vi "PicoScope6000aGetRapidBlockBulk.vi"(0 "handle in":i16, 1 "Acquisition Settings":T3 {"postTriggerSamples" format="%_6p"; "preTriggerSamples" format="%_6p"}, 2 "Buffer and Transfer Settings":T2 {"Down-Sample Mode" items=["None", "Aggregate", "Decimate", "Average"]; "Down Sample Ratio" step=1; "noOfSamples" format="%_6p"}, 3 "enabled array":i16[](array[numeric]), 7 "stop IsReady":bool, 11 "error in (no error)":errorcluster) -> (4 "handle out":i16, 6 "Buffers (Max or non-aggregated)":T1, 10 "Min Buffers":T1, 12 "noOfSamples":u64, 13 "nMaxSamples":u64, 14 "overflow":i16[](array[numeric]) format="%08b", 15 "error out":errorcluster)   [LabVIEW 2009]
doc: "This VI gets a set of blocks captured using rapid block mode. It outputs two-dimensional arrays for each channel that contain data from all the requested captures."
uses:
  ps6000a.dll
panel:
  in  "PicoAction 2":u32(ring) items=["NONE", "CLEAR_ALL", "ADD", "CLEAR_THIS_DATA_BUFFER", "CLEAR_WAVEFORM_DATA_BUFFERS", "CLEAR_WAVEFORM_READ_DATA_BUFFERS"]
  in  "PicoAction 1":u32(ring) items=["NONE", "CLEAR_ALL", "ADD", "CLEAR_THIS_DATA_BUFFER", "CLEAR_WAVEFORM_DATA_BUFFERS", "CLEAR_WAVEFORM_READ_DATA_BUFFERS"]
  # "Pico Buffer Actions"
  # "Samples can be equal to or less\nTotal Pre and Post Trigger Samples"
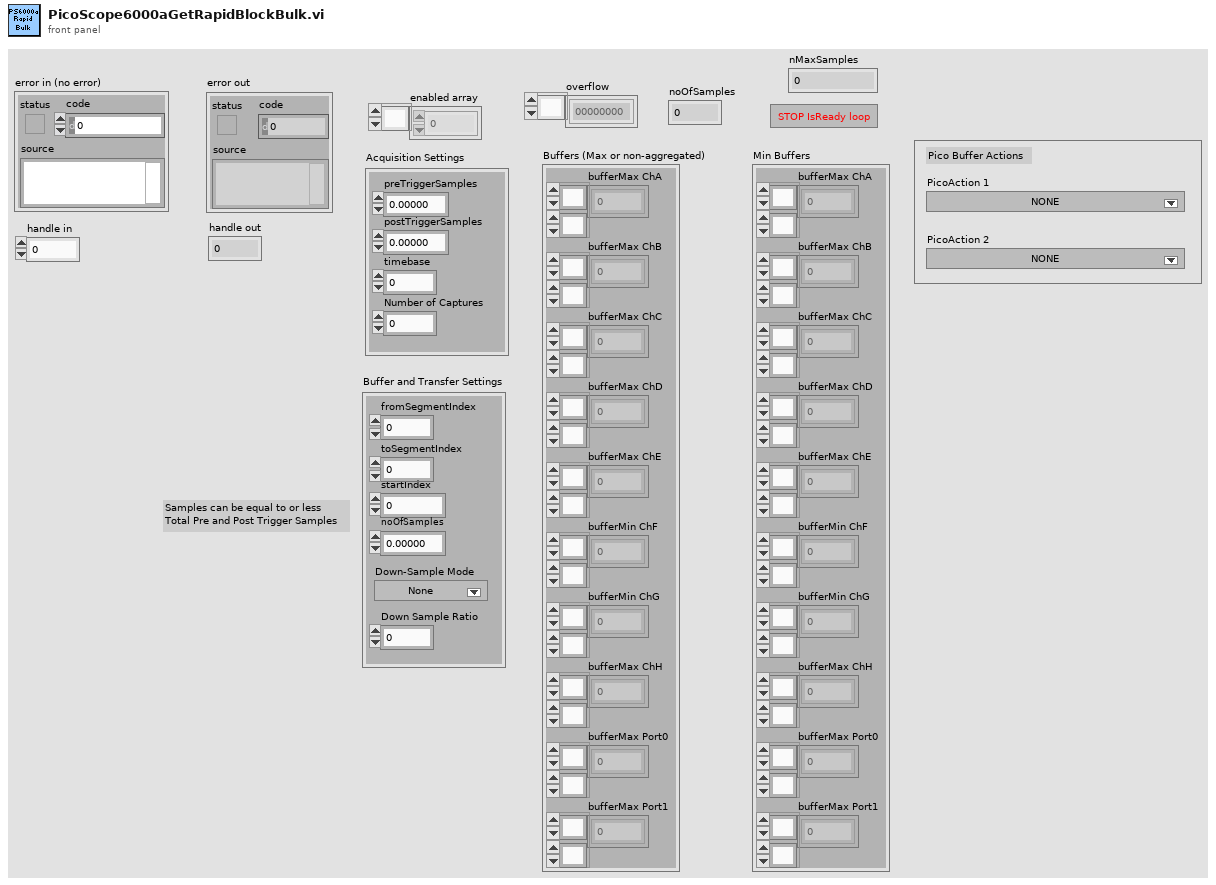
[diagram p1: front panel]
types:
  T1 = cluster{"bufferMax ChA":i16[][], "bufferMax ChB":i16[][], "bufferMax ChC":i16[][], "bufferMax ChD":i16[][], "bufferMax ChE":i16[][], "bufferMin ChF":i16[][], "bufferMin ChG":i16[][], "bufferMax ChH":i16[][], "bufferMax Port0":i16[][], "bufferMax Port1":i16[][]}
  T2 = cluster{"fromSegmentIndex":u64, "toSegmentIndex":u64, "startIndex":u64, "noOfSamples":u64, "Down-Sample Mode":u32, "Down Sample Ratio":u64}
  T3 = cluster{"preTriggerSamples":u64, "postTriggerSamples":u64, "timebase":u32, "Number of Captures":u64}
  T4 = enum32{"PICO_INT8_T", "PICO_INT16_T", "PICO_INT32_T", "PICO_UINT32_T", "PICO_INT64_T", ""}
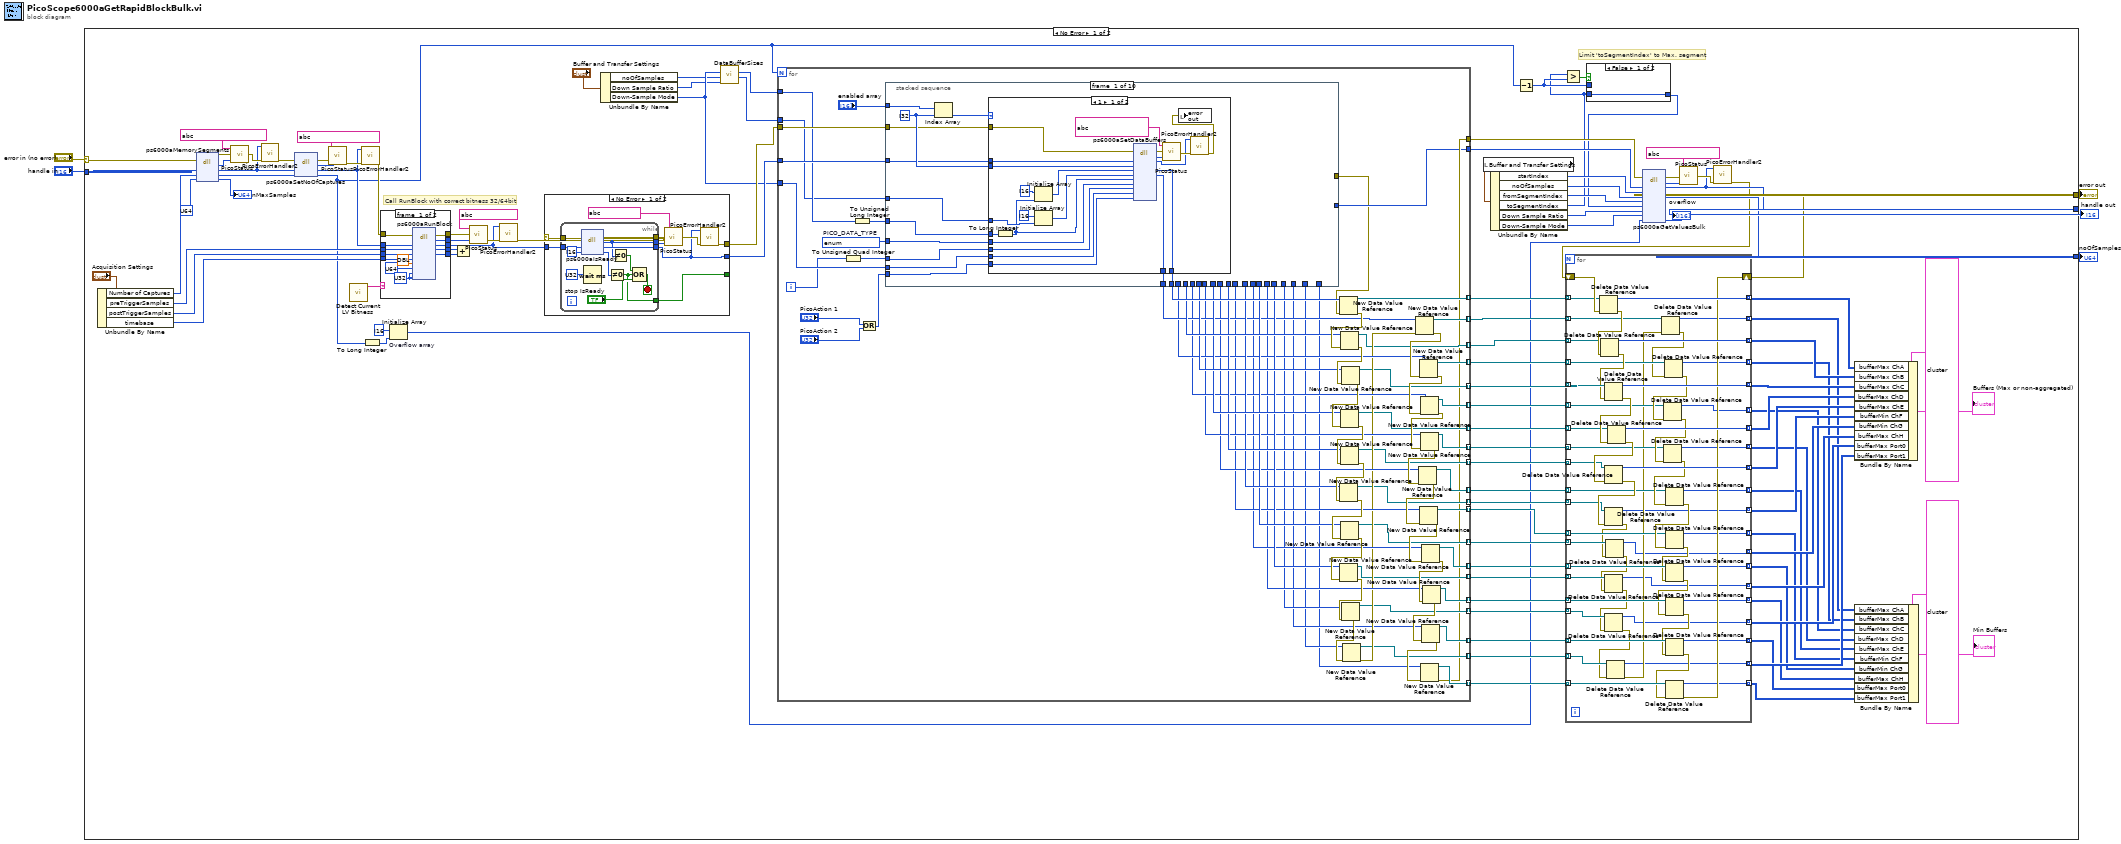
[diagram p0: block diagram]
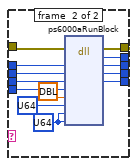
[diagram p2: hidden frame]
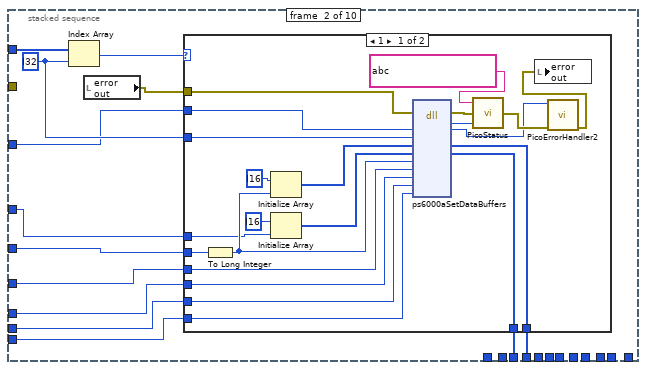
[diagram p5: hidden frame]
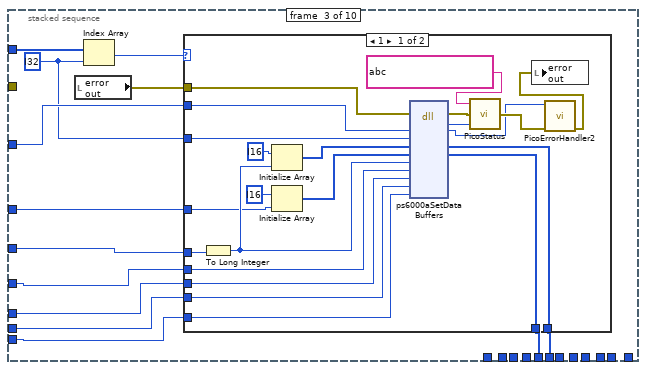
[diagram p7: hidden frame]
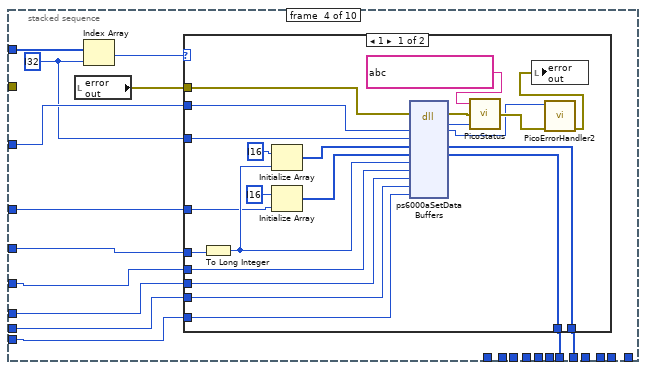
[diagram p9: hidden frame]
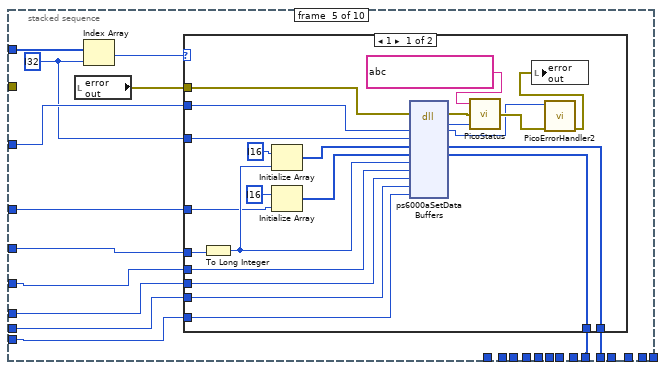
[diagram p11: hidden frame]
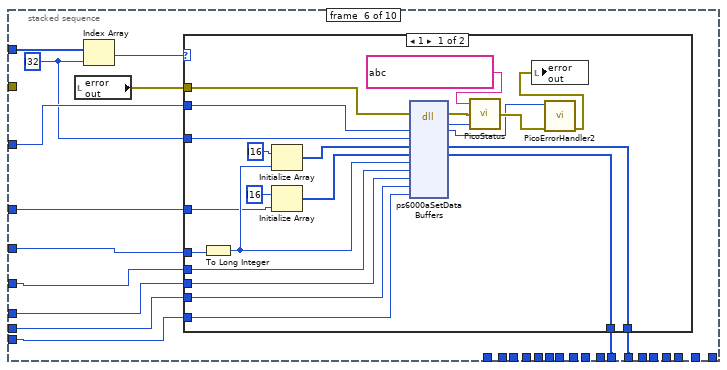
[diagram p13: hidden frame]
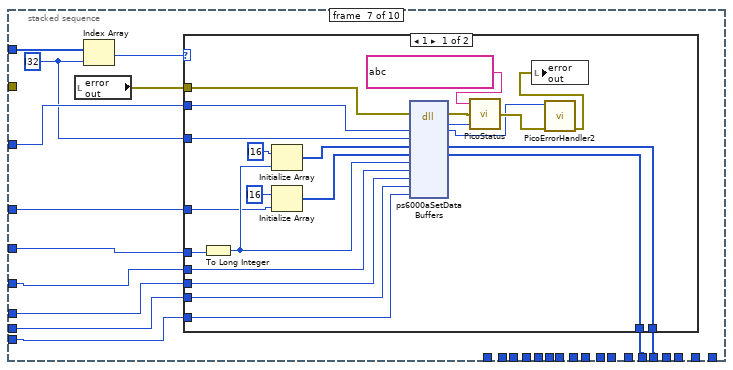
[diagram p15: hidden frame]
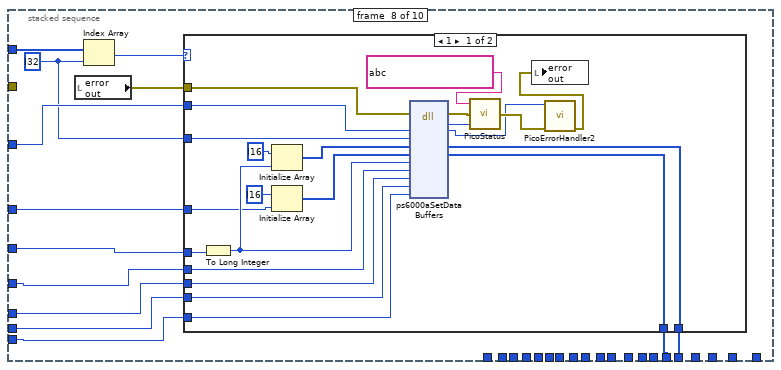
[diagram p17: hidden frame]
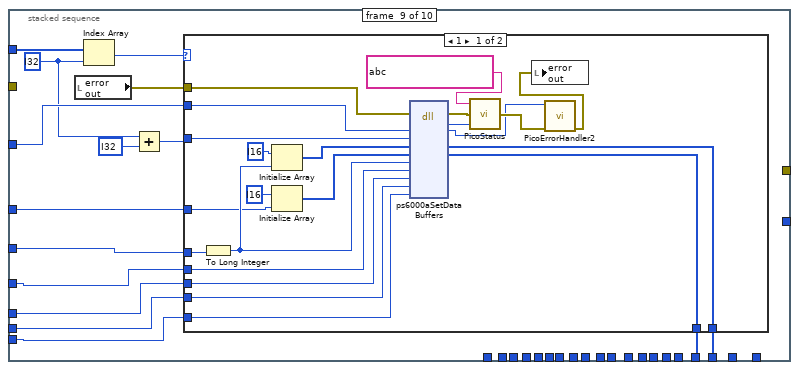
[diagram p19: hidden frame]
diagram:
  n1 = case shown="No Error" "error in (no error)" {
    selector: "error in (no error)" -> [w79 w662]
    tunnel: [w53 w662] -> w5
    tunnel: "handle in" -> [w78 w661]
    tunnel: [w75 w661] -> w4
    tunnel: [w103 u32 ? ("noOfSamples")] -> w1
    frame #0 {
      # "Call RunBlock with correct bitness 32/64bit"
      # "Limit 'toSegmentIndex' to Max. segment"
      n2 = Unbundle By Name("Acquisition Settings") -> ("Number of Captures"=w80:u64, "preTriggerSamples"=w107:u64, "postTriggerSamples"=w106:u64, "timebase"=w105:u32)
      n3 = dll-call lib="ps6000a.dll" fn="ps6000aMemorySegments" ("ps3000.dll:_ps3000_open_unit@0")(error in=w79, "handle"=w78, "nSegments"=w80, "nMaxSamples"=u64 ?) -> (error out=w91:errorcluster, "PICO_STATUS"=w92:u32, "handle"=w84:i16, "nSegments"=w88:u64, "nMaxSamples"=→"nMaxSamples":u64)  [unwired: 2 in, 1 out]
      n4 = call "PicoStatus.vi"("PICO STATUS"=w92, "error in"=w91, "source"=string ?) -> ("error out"=w85:errorcluster)
      n5 = call "PicoErrorHandler2.vi"("error in (no error)"=w85, "handle In"=w84) -> ("error out"=w11:errorcluster)  [unwired: 9 in]
      n6 = dll-call lib="ps6000a.dll" fn="ps6000aSetNoOfCaptures" ("ps3000.dll:_ps3000_open_unit@0")(error in=w11, "handle"=w84, "nCaptures"=w88) -> (error out=w87:errorcluster, "PICO_STATUS"=w82:u32, "handle"=w76:i16, "nCaptures"=w17:u64)  [unwired: 2 in, 1 out]
      n7 = call "PicoStatus.vi"("PICO STATUS"=w82, "error in"=w87, "source"=string ?) -> ("error out"=w83:errorcluster)
      n8 = call "Detect Current LV Bitness.vi"() -> ("bitness"=w12:string)  [unwired: 11 in]
      n9 = call "PicoErrorHandler2.vi"("error in (no error)"=w83, "handle In"=w76) -> ("error out"=w77:errorcluster)  [unwired: 9 in]
      n10 = To Long Integer(number=w17) -> (32bit integer=w25:i32)
      n11 = case shown="\"64\"" w12 {
        tunnel: [w126 w139] -> w113
        tunnel: [w125 w138] -> w112
        tunnel: [w124 w137] -> w110
        tunnel: [w123 w136] -> w109
        tunnel: w107 -> [w121 w134]
        tunnel: w106 -> [w120 w133]
        tunnel: w105 -> [w119 w132]
        tunnel: [w118 w131] -> w99
        tunnel: w77 -> [w116 w129]
        tunnel: w76 -> [w115 w128]
        frame #0 {
          w117 = u32 ? ("pParameter")
          n12 = dll-call lib="ps6000a.dll" fn="ps6000aRunBlock" ("ps3000.dll:_ps3000_open_unit@0")(error in=w116, "handle"=w115, "noOfPreTriggerSamples"=w121, "noOfPostTriggerSamples"=w120, "timebase"=w119, "timeIndisposedMs"=dbl ? ("pParameter"), "segmentIndex"=u64 ?, "lpReady"=w117, "pParameter"=w117) -> (error out=w123:errorcluster, "PICO_STATUS"=w124:u32, "handle"=w118:i16, "noOfPreTriggerSamples"=w126:u64, "noOfPostTriggerSamples"=w125:u64)  [unwired: 7 in, 1 out]
        }
        frame #1 {
          w130 = u64 ? ("pParameter")
          n13 = dll-call lib="ps6000a.dll" fn="ps6000aRunBlock" ("ps3000.dll:_ps3000_open_unit@0")(error in=w129, "handle"=w128, "noOfPreTriggerSamples"=w134, "noOfPostTriggerSamples"=w133, "timebase"=w132, "timeIndisposedMs"=dbl ? ("pParameter"), "segmentIndex"=u64 ?, "lpReady"=w130, "pParameter"=w130) -> (error out=w136:errorcluster, "PICO_STATUS"=w137:u32, "handle"=w131:i16, "noOfPreTriggerSamples"=w139:u64, "noOfPostTriggerSamples"=w138:u64)  [unwired: 7 in, 1 out]
        }
      }
      n14 = Initialize Array "Overflow array"(i16 ? ("element"), w25) -> (w24:i16[])
      n15 = Add(x=w113, y=w112) -> ()  [unwired: 1 out]
      n16 = call "PicoStatus.vi"("PICO STATUS"=w110, "error in"=w109, "source"=string ?) -> ("error out"=w104:errorcluster)
      n17 = call "PicoErrorHandler2.vi"("error in (no error)"=w104, "handle In"=w99) -> ("error out"=w102:errorcluster)  [unwired: 9 in]
      n18 = case shown="No Error" w102 {
        selector: w102 -> [w643 w658]
        tunnel: w99 -> [w644 w659]
        tunnel: [w637 w659] -> w100
        tunnel: [w638 w658] -> w101
        tunnel: [w636 bool ?] -> _
        frame #0 {
          n19 = while {
            tunnel: [w656] -> w637
            tunnel: w644 -> [w655]
            tunnel: [w652] -> w641
            tunnel: w643 -> [w651]
            tunnel: [w650] -> w642
            tunnel: [w645] -> w636
            stop <- w654 stop-if-true
            n20 = dll-call lib="ps6000a.dll" fn="ps6000aIsReady" ("ps3000.dll:_ps3000_open_unit@0")(error in=w651, "handle"=w655, "ready"=i16 ?) -> (error out=w650:errorcluster, "PICO_STATUS"=w652:u32, "handle"=w656:i16, "ready"=w646:i16)  [unwired: 2 in, 1 out]
            n21 = Wait (ms)(milliseconds to wait=u32 ?) -> ()  [unwired: 1 out]
            n22 = Not Equal To 0?(x=w646) -> (x != 0?=w645:bool)
            n23 = Not Equal To 0?(x=w652) -> (x != 0?=w653:bool)
            n24 = Compound Arithmetic op=OR(w653, w645, "stop IsReady") -> (w654:bool)
          }
          n25 = call "PicoStatus.vi"("PICO STATUS"=w641, "error in"=w642, "source"=string ?) -> ("error out"=w639:errorcluster)
          n26 = call "PicoErrorHandler2.vi"("error in (no error)"=w639, "handle In"=w637) -> ("error out"=w638:errorcluster)  [unwired: 9 in]
        }
        frame #1 {
        }
      }
      n27 = Unbundle By Name("Buffer and Transfer Settings") -> ("noOfSamples"=w8:u64, "Down Sample Ratio"=w9:u64, "Down-Sample Mode"=w10:u32)
      n28 = call "DataBufferSizes.vi"("Down Sample Ratio"=w9, "Number of Samples"=w8, "Down-Sample Mode"=w10) -> ("min Buffer Size"=w7:i32, "Max Buffer Size"=w6:i32)  [unwired: 7 in]
      n29 = for {
        N: w17 -> [_]
        tunnel: w101 -> [w277]
        tunnel: w100 -> [w276]
        tunnel: w10 -> [w275]
        tunnel: w6 -> [w274]
        tunnel: w7 -> [w273]
        tunnel: [w225] -> w74 mode=indexing
        tunnel: [w224] -> w73 mode=indexing
        tunnel: [w223] -> w72 mode=indexing
        tunnel: [w222] -> w71 mode=indexing
        tunnel: [w221] -> w70 mode=indexing
        tunnel: [w220] -> w69 mode=indexing
        tunnel: [w219] -> w68 mode=indexing
        tunnel: [w218] -> w67 mode=indexing
        tunnel: [w217] -> w66 mode=indexing
        tunnel: [w216] -> w65 mode=indexing
        tunnel: [w215] -> w64 mode=indexing
        tunnel: [w214] -> w63 mode=indexing
        tunnel: [w213] -> w62 mode=indexing
        tunnel: [w212] -> w61 mode=indexing
        tunnel: [w211] -> w60 mode=indexing
        tunnel: [w210] -> w59 mode=indexing
        tunnel: [w209] -> w58 mode=indexing
        tunnel: [w208] -> w57 mode=indexing
        tunnel: [w207] -> w56 mode=indexing
        tunnel: [w206] -> w55 mode=indexing
        tunnel: [w205] -> w54
        tunnel: [w204] -> w51
        i -> [w227]
        w267 = T4 ?  # PICO_DATA_TYPE
        n30 = To Unsigned Quad Integer(1:w227) -> (0:w226:u64)
        n31 = To Unsigned Long Integer(number=w274) -> (unsigned 32bit integer=w271:u32)
        n32 = Or(x="PicoAction 1", y="PicoAction 2") -> (x .or. y?=w268:u32)
        n33 = stacked-sequence {
          tunnel: "enabled array" -> [w289 w323 w359 w394 w429 w464 w499 w534 w571 w610]
          tunnel: w277 -> [w287 _ _ _ _ _ _ _ _ _]
          tunnel: w276 -> [w286 w322 w358 w393 w428 w463 w498 w533 w570 w609]
          tunnel: w271 -> [w285 w321 w349 w386 w421 w456 w491 w526 w564 w603]
          tunnel: w275 -> [w284 w315 w352 w389 w424 w459 w494 w529 w567 w606]
          tunnel: [w283 _ _ _ _ _ _ _ _ _] -> w240
          tunnel: [w282 _ _ _ _ _ _ _ _ _] -> w258
          tunnel: [_ w320 _ _ _ _ _ _ _ _] -> w239
          tunnel: [_ w319 _ _ _ _ _ _ _ _] -> w257
          tunnel: [_ _ w356 _ _ _ _ _ _ _] -> w238
          tunnel: [_ _ w355 _ _ _ _ _ _ _] -> w256
          tunnel: [_ _ _ w384 _ _ _ _ _ _] -> w237
          tunnel: [_ _ _ w383 _ _ _ _ _ _] -> w255
          tunnel: w267 -> [w281 w316 w350 w387 w422 w457 w492 w527 w565 w604]
          tunnel: w226 -> [w280 w314 w351 w388 w423 w458 w493 w528 w566 w605]
          tunnel: w268 -> [w279 w317 w353 w390 w425 w460 w495 w530 w568 w607]
          tunnel: [_ _ _ _ w418 _ _ _ _ _] -> w254
          tunnel: [_ _ _ _ _ _ _ w523 _ _] -> w250
          tunnel: [_ _ _ _ _ _ w488 _ _ _] -> w251
          tunnel: [_ _ _ _ _ w453 _ _ _ _] -> w253
          tunnel: [_ _ _ _ _ _ _ _ _ w601] -> w203
          tunnel: [_ _ _ _ _ _ _ _ _ w600] -> w204
          tunnel: [_ _ _ _ _ _ _ w524 _ _] -> w233
          tunnel: [_ _ _ _ _ _ w489 _ _ _] -> w234
          tunnel: [_ _ _ _ _ w454 _ _ _ _] -> w235
          tunnel: [_ _ _ _ w419 _ _ _ _ _] -> w236
          tunnel: w273 -> [w278 w313 w348 w385 w420 w455 w490 w525 w563 w602]
          tunnel: [_ _ _ _ _ _ _ _ w559 _] -> w231
          tunnel: [_ _ _ _ _ _ _ _ w558 _] -> w230
          tunnel: [_ _ _ _ _ _ _ _ _ w596] -> w229
          tunnel: [_ _ _ _ _ _ _ _ _ w595] -> w228
          frame #0 {
            w290 = i32 ? ("dimension size")
            n34 = Index Array(array=w289, index=w290) -> (element=w288:i16)
            n35 = case shown="1" w288 {
              tunnel: w290 -> [w307 _]
              tunnel: w287 -> [w312 _]
              tunnel: w286 -> [w309 _]
              tunnel: w285 -> [w292 _]
              tunnel: w284 -> [w301 _]
              tunnel: [w306 _] -> w283
              tunnel: [w305 _] -> w282
              tunnel: w281 -> [w300 _]
              tunnel: w280 -> [w299 _]
              tunnel: w279 -> [w298 _]
              tunnel: w278 -> [w294 _]
              frame #0 {
                n36 = To Long Integer(number=w292) -> (32bit integer=w291:i32)
                n37 = Initialize Array(i16 ? ("element"), w291) -> (w295:i16[])
                n38 = Initialize Array(i16 ? ("element"), w294) -> (w293:i16[])
                n39 = dll-call lib="ps6000a.dll" fn="ps6000aSetDataBuffers" ("ps3000.dll:_ps3000_open_unit@0")(error in=w312, "handle"=w309, "channel"=w307, "bufferMax"=w295, "bufferMin"=w293, "nSamples"=w291, "dataType"=w300, "waveform"=w299, "downSampleRatioMode"=w301, "action"=w298) -> (error out=w311:errorcluster, "PICO_STATUS"=w310:u32, "handle"=w302:i16, "bufferMax"=w305:i16[], "bufferMin"=w306:i16[])  [unwired: 8 in, 1 out]
                n40 = call "PicoStatus.vi"("PICO STATUS"=w310, "error in"=w311, "source"=string ?) -> ("error out"=w304:errorcluster)
                n41 = call "PicoErrorHandler2.vi"("error in (no error)"=w304, "handle In"=w302) -> ("error out"=w303:errorcluster)  [unwired: 9 in]
                n42 = local write "error out"(w303) -> ()
              }
              frame #1 {
              }
            }
          }
          frame #1 {
            w325 = i32 ? ("dimension size")
            n43 = Index Array(array=w323, index=w325) -> (element=w324:i16)
            n44 = local read "error out"() -> (w318:errorcluster)
            n45 = case shown="1" w324 {
              tunnel: w325 -> [w327 _]
              tunnel: w318 -> [w341 _]
              tunnel: w322 -> [w326 _]
              tunnel: w314 -> [w336 _]
              tunnel: w321 -> [w331 _]
              tunnel: [w339 _] -> w320
              tunnel: [w340 _] -> w319
              tunnel: w317 -> [w338 _]
              tunnel: w316 -> [w335 _]
              tunnel: w315 -> [w337 _]
              tunnel: w313 -> [w330 _]
              frame #0 {
                n46 = To Long Integer(number=w331) -> (32bit integer=w332:i32)
                n47 = Initialize Array(i16 ? ("element"), w332) -> (w328:i16[])
                n48 = Initialize Array(i16 ? ("element"), w330) -> (w329:i16[])
                n49 = dll-call lib="ps6000a.dll" fn="ps6000aSetDataBuffers" ("ps3000.dll:_ps3000_open_unit@0")(error in=w341, "handle"=w326, "channel"=w327, "bufferMax"=w328, "bufferMin"=w329, "nSamples"=w332, "dataType"=w335, "waveform"=w336, "downSampleRatioMode"=w337, "action"=w338) -> (error out=w344:errorcluster, "PICO_STATUS"=w343:u32, "handle"=w342:i16, "bufferMax"=w340:i16[], "bufferMin"=w339:i16[])  [unwired: 8 in, 1 out]
                n50 = call "PicoStatus.vi"("PICO STATUS"=w343, "error in"=w344, "source"=string ?) -> ("error out"=w346:errorcluster)
                n51 = call "PicoErrorHandler2.vi"("error in (no error)"=w346, "handle In"=w342) -> ("error out"=w345:errorcluster)  [unwired: 9 in]
                n52 = local write "error out"(w345) -> ()
              }
              frame #1 {
              }
            }
          }
          frame #2 {
            w354 = i32 ? ("dimension size")
            n53 = local read "error out"() -> (w357:errorcluster)
            n54 = Index Array(array=w359, index=w354) -> (element=w360:i16)
            n55 = case shown="1" w360 {
              tunnel: w357 -> [w374 _]
              tunnel: w358 -> [w373 _]
              tunnel: [w375 _] -> w356
              tunnel: [w376 _] -> w355
              tunnel: w354 -> [w372 _]
              tunnel: w353 -> [w367 _]
              tunnel: w352 -> [w366 _]
              tunnel: w351 -> [w365 _]
              tunnel: w350 -> [w364 _]
              tunnel: w349 -> [w363 _]
              tunnel: w348 -> [w361 _]
              frame #0 {
                n56 = To Long Integer(number=w363) -> (32bit integer=w362:i32)
                n57 = Initialize Array(i16 ? ("element"), w362) -> (w369:i16[])
                n58 = Initialize Array(i16 ? ("element"), w361) -> (w368:i16[])
                n59 = dll-call lib="ps6000a.dll" fn="ps6000aSetDataBuffers" ("ps3000.dll:_ps3000_open_unit@0")(error in=w374, "handle"=w373, "channel"=w372, "bufferMax"=w369, "bufferMin"=w368, "nSamples"=w362, "dataType"=w364, "waveform"=w365, "downSampleRatioMode"=w366, "action"=w367) -> (error out=w379:errorcluster, "PICO_STATUS"=w378:u32, "handle"=w377:i16, "bufferMax"=w376:i16[], "bufferMin"=w375:i16[])  [unwired: 8 in, 1 out]
                n60 = call "PicoStatus.vi"("PICO STATUS"=w378, "error in"=w379, "source"=string ?) -> ("error out"=w381:errorcluster)
                n61 = call "PicoErrorHandler2.vi"("error in (no error)"=w381, "handle In"=w377) -> ("error out"=w380:errorcluster)  [unwired: 9 in]
                n62 = local write "error out"(w380) -> ()
              }
              frame #1 {
              }
            }
          }
          frame #3 {
            w391 = i32 ? ("dimension size")
            n63 = local read "error out"() -> (w392:errorcluster)
            n64 = Index Array(array=w394, index=w391) -> (element=w395:i16)
            n65 = case shown="1" w395 {
              tunnel: w392 -> [w409 _]
              tunnel: w393 -> [w408 _]
              tunnel: [w410 _] -> w384
              tunnel: [w411 _] -> w383
              tunnel: w391 -> [w407 _]
              tunnel: w390 -> [w402 _]
              tunnel: w389 -> [w401 _]
              tunnel: w388 -> [w400 _]
              tunnel: w387 -> [w399 _]
              tunnel: w386 -> [w398 _]
              tunnel: w385 -> [w396 _]
              frame #0 {
                n66 = To Long Integer(number=w398) -> (32bit integer=w397:i32)
                n67 = Initialize Array(i16 ? ("element"), w397) -> (w404:i16[])
                n68 = Initialize Array(i16 ? ("element"), w396) -> (w403:i16[])
                n69 = dll-call lib="ps6000a.dll" fn="ps6000aSetDataBuffers" ("ps3000.dll:_ps3000_open_unit@0")(error in=w409, "handle"=w408, "channel"=w407, "bufferMax"=w404, "bufferMin"=w403, "nSamples"=w397, "dataType"=w399, "waveform"=w400, "downSampleRatioMode"=w401, "action"=w402) -> (error out=w414:errorcluster, "PICO_STATUS"=w413:u32, "handle"=w412:i16, "bufferMax"=w411:i16[], "bufferMin"=w410:i16[])  [unwired: 8 in, 1 out]
                n70 = call "PicoStatus.vi"("PICO STATUS"=w413, "error in"=w414, "source"=string ?) -> ("error out"=w416:errorcluster)
                n71 = call "PicoErrorHandler2.vi"("error in (no error)"=w416, "handle In"=w412) -> ("error out"=w415:errorcluster)  [unwired: 9 in]
                n72 = local write "error out"(w415) -> ()
              }
              frame #1 {
              }
            }
          }
          frame #4 {
            w426 = i32 ? ("dimension size")
            n73 = local read "error out"() -> (w427:errorcluster)
            n74 = Index Array(array=w429, index=w426) -> (element=w430:i16)
            n75 = case shown="1" w430 {
              tunnel: w427 -> [w444 _]
              tunnel: w428 -> [w443 _]
              tunnel: [w445 _] -> w419
              tunnel: [w446 _] -> w418
              tunnel: w426 -> [w442 _]
              tunnel: w425 -> [w437 _]
              tunnel: w424 -> [w436 _]
              tunnel: w423 -> [w435 _]
              tunnel: w422 -> [w434 _]
              tunnel: w421 -> [w433 _]
              tunnel: w420 -> [w431 _]
              frame #0 {
                n76 = To Long Integer(number=w433) -> (32bit integer=w432:i32)
                n77 = Initialize Array(i16 ? ("element"), w432) -> (w439:i16[])
                n78 = Initialize Array(i16 ? ("element"), w431) -> (w438:i16[])
                n79 = dll-call lib="ps6000a.dll" fn="ps6000aSetDataBuffers" ("ps3000.dll:_ps3000_open_unit@0")(error in=w444, "handle"=w443, "channel"=w442, "bufferMax"=w439, "bufferMin"=w438, "nSamples"=w432, "dataType"=w434, "waveform"=w435, "downSampleRatioMode"=w436, "action"=w437) -> (error out=w449:errorcluster, "PICO_STATUS"=w448:u32, "handle"=w447:i16, "bufferMax"=w446:i16[], "bufferMin"=w445:i16[])  [unwired: 8 in, 1 out]
                n80 = call "PicoStatus.vi"("PICO STATUS"=w448, "error in"=w449, "source"=string ?) -> ("error out"=w451:errorcluster)
                n81 = call "PicoErrorHandler2.vi"("error in (no error)"=w451, "handle In"=w447) -> ("error out"=w450:errorcluster)  [unwired: 9 in]
                n82 = local write "error out"(w450) -> ()
              }
              frame #1 {
              }
            }
          }
          frame #5 {
            w461 = i32 ? ("dimension size")
            n83 = local read "error out"() -> (w462:errorcluster)
            n84 = Index Array(array=w464, index=w461) -> (element=w465:i16)
            n85 = case shown="1" w465 {
              tunnel: w462 -> [w479 _]
              tunnel: w463 -> [w478 _]
              tunnel: [w480 _] -> w454
              tunnel: [w481 _] -> w453
              tunnel: w461 -> [w477 _]
              tunnel: w460 -> [w472 _]
              tunnel: w459 -> [w471 _]
              tunnel: w458 -> [w470 _]
              tunnel: w457 -> [w469 _]
              tunnel: w456 -> [w468 _]
              tunnel: w455 -> [w466 _]
              frame #0 {
                n86 = To Long Integer(number=w468) -> (32bit integer=w467:i32)
                n87 = Initialize Array(i16 ? ("element"), w467) -> (w474:i16[])
                n88 = Initialize Array(i16 ? ("element"), w466) -> (w473:i16[])
                n89 = dll-call lib="ps6000a.dll" fn="ps6000aSetDataBuffers" ("ps3000.dll:_ps3000_open_unit@0")(error in=w479, "handle"=w478, "channel"=w477, "bufferMax"=w474, "bufferMin"=w473, "nSamples"=w467, "dataType"=w469, "waveform"=w470, "downSampleRatioMode"=w471, "action"=w472) -> (error out=w484:errorcluster, "PICO_STATUS"=w483:u32, "handle"=w482:i16, "bufferMax"=w481:i16[], "bufferMin"=w480:i16[])  [unwired: 8 in, 1 out]
                n90 = call "PicoStatus.vi"("PICO STATUS"=w483, "error in"=w484, "source"=string ?) -> ("error out"=w486:errorcluster)
                n91 = call "PicoErrorHandler2.vi"("error in (no error)"=w486, "handle In"=w482) -> ("error out"=w485:errorcluster)  [unwired: 9 in]
                n92 = local write "error out"(w485) -> ()
              }
              frame #1 {
              }
            }
          }
          frame #6 {
            w496 = i32 ? ("dimension size")
            n93 = local read "error out"() -> (w497:errorcluster)
            n94 = Index Array(array=w499, index=w496) -> (element=w500:i16)
            n95 = case shown="1" w500 {
              tunnel: w497 -> [w514 _]
              tunnel: w498 -> [w513 _]
              tunnel: [w515 _] -> w489
              tunnel: [w516 _] -> w488
              tunnel: w496 -> [w512 _]
              tunnel: w495 -> [w507 _]
              tunnel: w494 -> [w506 _]
              tunnel: w493 -> [w505 _]
              tunnel: w492 -> [w504 _]
              tunnel: w491 -> [w503 _]
              tunnel: w490 -> [w501 _]
              frame #0 {
                n96 = To Long Integer(number=w503) -> (32bit integer=w502:i32)
                n97 = Initialize Array(i16 ? ("element"), w502) -> (w509:i16[])
                n98 = Initialize Array(i16 ? ("element"), w501) -> (w508:i16[])
                n99 = dll-call lib="ps6000a.dll" fn="ps6000aSetDataBuffers" ("ps3000.dll:_ps3000_open_unit@0")(error in=w514, "handle"=w513, "channel"=w512, "bufferMax"=w509, "bufferMin"=w508, "nSamples"=w502, "dataType"=w504, "waveform"=w505, "downSampleRatioMode"=w506, "action"=w507) -> (error out=w519:errorcluster, "PICO_STATUS"=w518:u32, "handle"=w517:i16, "bufferMax"=w516:i16[], "bufferMin"=w515:i16[])  [unwired: 8 in, 1 out]
                n100 = call "PicoStatus.vi"("PICO STATUS"=w518, "error in"=w519, "source"=string ?) -> ("error out"=w521:errorcluster)
                n101 = call "PicoErrorHandler2.vi"("error in (no error)"=w521, "handle In"=w517) -> ("error out"=w520:errorcluster)  [unwired: 9 in]
                n102 = local write "error out"(w520) -> ()
              }
              frame #1 {
              }
            }
          }
          frame #7 {
            w531 = i32 ? ("dimension size")
            n103 = local read "error out"() -> (w532:errorcluster)
            n104 = Index Array(array=w534, index=w531) -> (element=w535:i16)
            n105 = case shown="1" w535 {
              tunnel: w532 -> [w549 _]
              tunnel: w533 -> [w548 _]
              tunnel: [w550 _] -> w524
              tunnel: [w551 _] -> w523
              tunnel: w531 -> [w547 _]
              tunnel: w530 -> [w542 _]
              tunnel: w529 -> [w541 _]
              tunnel: w528 -> [w540 _]
              tunnel: w527 -> [w539 _]
              tunnel: w526 -> [w538 _]
              tunnel: w525 -> [w536 _]
              frame #0 {
                n106 = To Long Integer(number=w538) -> (32bit integer=w537:i32)
                n107 = Initialize Array(i16 ? ("element"), w537) -> (w544:i16[])
                n108 = Initialize Array(i16 ? ("element"), w536) -> (w543:i16[])
                n109 = dll-call lib="ps6000a.dll" fn="ps6000aSetDataBuffers" ("ps3000.dll:_ps3000_open_unit@0")(error in=w549, "handle"=w548, "channel"=w547, "bufferMax"=w544, "bufferMin"=w543, "nSamples"=w537, "dataType"=w539, "waveform"=w540, "downSampleRatioMode"=w541, "action"=w542) -> (error out=w554:errorcluster, "PICO_STATUS"=w553:u32, "handle"=w552:i16, "bufferMax"=w551:i16[], "bufferMin"=w550:i16[])  [unwired: 8 in, 1 out]
                n110 = call "PicoStatus.vi"("PICO STATUS"=w553, "error in"=w554, "source"=string ?) -> ("error out"=w556:errorcluster)
                n111 = call "PicoErrorHandler2.vi"("error in (no error)"=w556, "handle In"=w552) -> ("error out"=w555:errorcluster)  [unwired: 9 in]
                n112 = local write "error out"(w555) -> ()
              }
              frame #1 {
              }
            }
          }
          frame #8 {
            w562 = i32 ? ("dimension size")
            n113 = local read "error out"() -> (w569:errorcluster)
            n114 = Index Array(array=w571, index=w562) -> (element=w572:i16)
            n115 = Add(x=w562, y=i32 ?) -> (x+y=w561:i32)
            n116 = case shown="1" w572 {
              tunnel: w569 -> [w586 _]
              tunnel: w570 -> [w585 _]
              tunnel: [w587 _] -> w559
              tunnel: [w588 _] -> w558
              tunnel: w561 -> [w584 _]
              tunnel: w568 -> [w579 _]
              tunnel: w567 -> [w578 _]
              tunnel: w566 -> [w577 _]
              tunnel: w565 -> [w576 _]
              tunnel: w564 -> [w575 _]
              tunnel: w563 -> [w573 _]
              frame #0 {
                n117 = To Long Integer(number=w575) -> (32bit integer=w574:i32)
                n118 = Initialize Array(i16 ? ("element"), w574) -> (w581:i16[])
                n119 = Initialize Array(i16 ? ("element"), w573) -> (w580:i16[])
                n120 = dll-call lib="ps6000a.dll" fn="ps6000aSetDataBuffers" ("ps3000.dll:_ps3000_open_unit@0")(error in=w586, "handle"=w585, "channel"=w584, "bufferMax"=w581, "bufferMin"=w580, "nSamples"=w574, "dataType"=w576, "waveform"=w577, "downSampleRatioMode"=w578, "action"=w579) -> (error out=w591:errorcluster, "PICO_STATUS"=w590:u32, "handle"=w589:i16, "bufferMax"=w588:i16[], "bufferMin"=w587:i16[])  [unwired: 8 in, 1 out]
                n121 = call "PicoStatus.vi"("PICO STATUS"=w590, "error in"=w591, "source"=string ?) -> ("error out"=w593:errorcluster)
                n122 = call "PicoErrorHandler2.vi"("error in (no error)"=w593, "handle In"=w589) -> ("error out"=w592:errorcluster)  [unwired: 9 in]
                n123 = local write "error out"(w592) -> ()
              }
              frame #1 {
              }
            }
          }
          frame #9 {
            w597 = i32 ? ("dimension size")
            n124 = local read "error out"() -> (w608:errorcluster)
            n125 = Index Array(array=w610, index=w597) -> (element=w611:i16)
            n126 = Add(x=w597, y=i32 ?) -> (x+y=w598:i32)
            n127 = case shown="1" w611 {
              tunnel: w608 -> [w627 w635]
              tunnel: w609 -> [w626 w634]
              tunnel: [w628 _] -> w596
              tunnel: [w629 _] -> w595
              tunnel: w598 -> [w625 _]
              tunnel: w607 -> [w620 _]
              tunnel: w606 -> [w619 _]
              tunnel: w605 -> [w618 _]
              tunnel: w604 -> [w617 _]
              tunnel: w603 -> [w616 _]
              tunnel: w602 -> [w614 _]
              tunnel: [w613 w635] -> w601
              tunnel: [w612 w634] -> w600
              frame #0 {
                n128 = To Long Integer(number=w616) -> (32bit integer=w615:i32)
                n129 = Initialize Array(i16 ? ("element"), w615) -> (w622:i16[])
                n130 = Initialize Array(i16 ? ("element"), w614) -> (w621:i16[])
                n131 = dll-call lib="ps6000a.dll" fn="ps6000aSetDataBuffers" ("ps3000.dll:_ps3000_open_unit@0")(error in=w627, "handle"=w626, "channel"=w625, "bufferMax"=w622, "bufferMin"=w621, "nSamples"=w615, "dataType"=w617, "waveform"=w618, "downSampleRatioMode"=w619, "action"=w620) -> (error out=w631:errorcluster, "PICO_STATUS"=w630:u32, "handle"=w612:i16, "bufferMax"=w629:i16[], "bufferMin"=w628:i16[])  [unwired: 8 in, 1 out]
                n132 = call "PicoStatus.vi"("PICO STATUS"=w630, "error in"=w631, "source"=string ?) -> ("error out"=w632:errorcluster)
                n133 = call "PicoErrorHandler2.vi"("error in (no error)"=w632, "handle In"=w612) -> ("error out"=w613:errorcluster)  [unwired: 9 in]
              }
              frame #1 {
              }
            }
          }
        }
        n134 = New Data Value Reference(data value=w258, error in=w203) -> (data value reference=w224:refnum<data-value>, error out=w263:errorcluster)
        n135 = New Data Value Reference(data value=w257, error in=w263) -> (data value reference=w223:refnum<data-value>, error out=w262:errorcluster)
        n136 = New Data Value Reference(data value=w256, error in=w262) -> (data value reference=w221:refnum<data-value>, error out=w266:errorcluster)
        n137 = New Data Value Reference(data value=w255, error in=w266) -> (data value reference=w219:refnum<data-value>, error out=w265:errorcluster)
        n138 = New Data Value Reference(data value=w254, error in=w265) -> (data value reference=w217:refnum<data-value>, error out=w264:errorcluster)
        n139 = New Data Value Reference(data value=w253, error in=w264) -> (data value reference=w215:refnum<data-value>, error out=w252:errorcluster)
        n140 = New Data Value Reference(data value=w251, error in=w252) -> (data value reference=w213:refnum<data-value>, error out=w260:errorcluster)
        n141 = New Data Value Reference(data value=w250, error in=w260) -> (data value reference=w211:refnum<data-value>, error out=w259:errorcluster)
        n142 = New Data Value Reference(data value=w231, error in=w259) -> (data value reference=w209:refnum<data-value>, error out=w261:errorcluster)
        n143 = New Data Value Reference(data value=w229, error in=w261) -> (data value reference=w207:refnum<data-value>, error out=w232:errorcluster)
        n144 = New Data Value Reference(data value=w240, error in=w232) -> (data value reference=w225:refnum<data-value>, error out=w246:errorcluster)
        n145 = New Data Value Reference(data value=w239, error in=w246) -> (data value reference=w222:refnum<data-value>, error out=w245:errorcluster)
        n146 = New Data Value Reference(data value=w238, error in=w245) -> (data value reference=w220:refnum<data-value>, error out=w249:errorcluster)
        n147 = New Data Value Reference(data value=w237, error in=w249) -> (data value reference=w218:refnum<data-value>, error out=w248:errorcluster)
        n148 = New Data Value Reference(data value=w236, error in=w248) -> (data value reference=w216:refnum<data-value>, error out=w247:errorcluster)
        n149 = New Data Value Reference(data value=w235, error in=w247) -> (data value reference=w214:refnum<data-value>, error out=w241:errorcluster)
        n150 = New Data Value Reference(data value=w234, error in=w241) -> (data value reference=w212:refnum<data-value>, error out=w243:errorcluster)
        n151 = New Data Value Reference(data value=w233, error in=w243) -> (data value reference=w210:refnum<data-value>, error out=w242:errorcluster)
        n152 = New Data Value Reference(data value=w230, error in=w242) -> (data value reference=w208:refnum<data-value>, error out=w244:errorcluster)
        n153 = New Data Value Reference(data value=w228, error in=w244) -> (data value reference=w206:refnum<data-value>, error out=w205:errorcluster)
      }
      n154 = local read "Buffer and Transfer Settings"() -> (w97:T2)
      n155 = Unbundle By Name(w97) -> ("startIndex"=w18:u64, "noOfSamples"=w22:u64, "fromSegmentIndex"=w21:u64, "toSegmentIndex"=w14:u64, "Down Sample Ratio"=w20:u64, "Down-Sample Mode"=w19:u32)
      n156 = Decrement(x=w17) -> (x-1=w15:u64)
      n157 = Greater?(x=w14, y=w15) -> (0:w13:bool)
      n158 = case shown="False" w13 {
        tunnel: [w140 w141] -> w16
        tunnel: w14 -> [w140 _]
        tunnel: w15 -> [_ w141]
        frame #0 {
        }
        frame #1 {
        }
      }
      n159 = dll-call lib="ps6000a.dll" fn="ps6000aGetValuesBulk" ("ps3000.dll:_ps3000_open_unit@0")(error in=w54, "handle"=w51, "startIndex"=w18, "noOfSamples"=w22, "fromSegmentIndex"=w21, "toSegmentIndex"=w16, "downSampleRatio"=w20, "downSampleRatioMode"=w19, "overflow"=w24) -> (error out=w95:errorcluster, "PICO_STATUS"=w94:u32, "handle"=w75:i16, "noOfSamples"=w103:u64, "overflow"=→"overflow":i16[])  [unwired: 7 in, 1 out]
      n160 = call "PicoStatus.vi"("PICO STATUS"=w94, "error in"=w95, "source"=string ?) -> ("error out"=w96:errorcluster)
      n161 = call "PicoErrorHandler2.vi"("error in (no error)"=w96, "handle In"=w75) -> ("error out"=w52:errorcluster)  [unwired: 9 in]
      n162 = for {
        shift-right: [w157] -> w53
        shift-left: w52 -> [w195]
        tunnel: w70 -> [w202] mode=indexing
        tunnel: [w198] -> w48 mode=indexing
        tunnel: [w197] -> w47 mode=indexing
        tunnel: [w196] -> w46 mode=indexing
        tunnel: w72 -> [w192] mode=indexing
        tunnel: w73 -> [w191] mode=indexing
        tunnel: [w190] -> w49 mode=indexing
        tunnel: [w189] -> w50 mode=indexing
        tunnel: w74 -> [w188] mode=indexing
        tunnel: w71 -> [w187] mode=indexing
        tunnel: w69 -> [w184] mode=indexing
        tunnel: w68 -> [w183] mode=indexing
        tunnel: w67 -> [w179] mode=indexing
        tunnel: w66 -> [w178] mode=indexing
        tunnel: w65 -> [w177] mode=indexing
        tunnel: w64 -> [w176] mode=indexing
        tunnel: w63 -> [w175] mode=indexing
        tunnel: w62 -> [w174] mode=indexing
        tunnel: w61 -> [w173] mode=indexing
        tunnel: w60 -> [w172] mode=indexing
        tunnel: w59 -> [w171] mode=indexing
        tunnel: w58 -> [w170] mode=indexing
        tunnel: w57 -> [w169] mode=indexing
        tunnel: w56 -> [w168] mode=indexing
        tunnel: w55 -> [w167] mode=indexing
        tunnel: [w156] -> w36 mode=indexing
        tunnel: [w155] -> w35 mode=indexing
        tunnel: [w154] -> w34 mode=indexing
        tunnel: [w153] -> w33 mode=indexing
        tunnel: [w152] -> w32 mode=indexing
        tunnel: [w151] -> w31 mode=indexing
        tunnel: [w150] -> w30 mode=indexing
        tunnel: [w149] -> w29 mode=indexing
        tunnel: [w148] -> w28 mode=indexing
        tunnel: [w147] -> w27 mode=indexing
        tunnel: [w146] -> w44 mode=indexing
        tunnel: [w145] -> w43 mode=indexing
        tunnel: [w144] -> w42 mode=indexing
        tunnel: [w143] -> w41 mode=indexing
        tunnel: [w142] -> w40 mode=indexing
        n163 = Delete Data Value Reference(data value reference=w191, error in=w195) -> (data value=w189:i16[], error out=w194:errorcluster)
        n164 = Delete Data Value Reference(data value reference=w192, error in=w194) -> (data value=w190:i16[], error out=w193:errorcluster)
        n165 = Delete Data Value Reference(data value reference=w202, error in=w193) -> (data value=w198:i16[], error out=w201:errorcluster)
        n166 = Delete Data Value Reference(data value reference=w183, error in=w201) -> (data value=w197:i16[], error out=w200:errorcluster)
        n167 = Delete Data Value Reference(data value reference=w178, error in=w200) -> (data value=w196:i16[], error out=w199:errorcluster)
        n168 = Delete Data Value Reference(data value reference=w176, error in=w199) -> (data value=w146:i16[], error out=w166:errorcluster)
        n169 = Delete Data Value Reference(data value reference=w174, error in=w166) -> (data value=w145:i16[], error out=w165:errorcluster)
        n170 = Delete Data Value Reference(data value reference=w172, error in=w165) -> (data value=w144:i16[], error out=w164:errorcluster)
        n171 = Delete Data Value Reference(data value reference=w170, error in=w164) -> (data value=w143:i16[], error out=w163:errorcluster)
        n172 = Delete Data Value Reference(data value reference=w168, error in=w163) -> (data value=w142:i16[], error out=w162:errorcluster)
        n173 = Delete Data Value Reference(data value reference=w188, error in=w162) -> (data value=w156:i16[], error out=w186:errorcluster)
        n174 = Delete Data Value Reference(data value reference=w187, error in=w186) -> (data value=w155:i16[], error out=w185:errorcluster)
        n175 = Delete Data Value Reference(data value reference=w184, error in=w185) -> (data value=w154:i16[], error out=w180:errorcluster)
        n176 = Delete Data Value Reference(data value reference=w179, error in=w180) -> (data value=w153:i16[], error out=w182:errorcluster)
        n177 = Delete Data Value Reference(data value reference=w177, error in=w182) -> (data value=w152:i16[], error out=w181:errorcluster)
        n178 = Delete Data Value Reference(data value reference=w175, error in=w181) -> (data value=w151:i16[], error out=w161:errorcluster)
        n179 = Delete Data Value Reference(data value reference=w173, error in=w161) -> (data value=w150:i16[], error out=w160:errorcluster)
        n180 = Delete Data Value Reference(data value reference=w171, error in=w160) -> (data value=w149:i16[], error out=w159:errorcluster)
        n181 = Delete Data Value Reference(data value reference=w169, error in=w159) -> (data value=w148:i16[], error out=w158:errorcluster)
        n182 = Delete Data Value Reference(data value reference=w167, error in=w158) -> (data value=w147:i16[], error out=w157:errorcluster)
      }
      n183 = Bundle By Name(cluster=T1 ?, "bufferMax ChA"=w50, "bufferMax ChB"=w49, "bufferMax ChC"=w48, "bufferMax ChD"=w47, "bufferMax ChE"=w46, "bufferMin ChF"=w44, "bufferMin ChG"=w43, "bufferMax ChH"=w42, "bufferMax Port0"=w41, "bufferMax Port1"=w40) -> (→"Buffers (Max or non-aggregated)":T1)
      n184 = Bundle By Name(cluster=T1 ?, "bufferMax ChA"=w36, "bufferMax ChB"=w35, "bufferMax ChC"=w34, "bufferMax ChD"=w33, "bufferMax ChE"=w32, "bufferMin ChF"=w31, "bufferMin ChG"=w30, "bufferMax ChH"=w29, "bufferMax Port0"=w28, "bufferMax Port1"=w27) -> (→"Min Buffers":T1)
    }
    frame #1 {
    }
  }
  "error out" <- w5
  "handle out" <- w4
  "noOfSamples" <- w1
